vi "SensorNicmos.vi"(0 "error in (no error)":errorcluster) -> (3 "error out":errorcluster, 5 "Intensity":dbl)   [LabVIEW 2009]
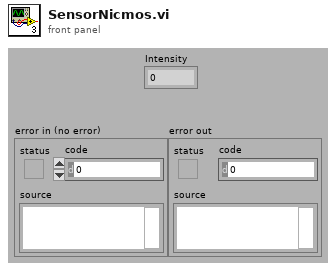
[diagram p1: front panel]
types:
  T1 = typedef "NICMOS.DATA.ctl" = cluster{"DATA":i32[][][], "INDEX":i32}
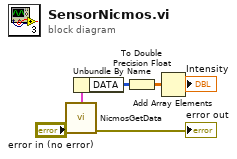
[diagram p0: block diagram]
diagram:
  n1 = call "NicmosGetData.vi"("error in (no error)"="error in (no error)") -> ("DATA"=w1:T1, "error out"=→"error out":errorcluster)  [unwired: 7 in]
  n2 = Unbundle By Name(w1) -> ("DATA"=w2:i32[][][])
  n3 = To Double Precision Float(number=w2) -> (double precision float=w3:dbl[][][])
  n4 = Add Array Elements(numeric array=w3) -> (sum=→"Intensity":dbl)
